vi "DQMH-GenNet Set Message Queue.vi"(8 "error in (no error)":errorcluster, 10 "Message Queue in":refnum<class "Delacor_lib_QMH_Message Queue.lvclass">, 11 "DQMH-GenNet Message Queue in":refnum<class "DQMH-GenNet Message Queue.lvclass">) -> (0 "error out":errorcluster, 3 "DQMH-GenNet Message Queue out":refnum<class "DQMH-GenNet Message Queue.lvclass">)   [LabVIEW 2014, in "hse-gennet.lvlib" / "DQMH-GenNet Message Queue.lvclass"]
doc: "Gets the message queue from the original DQMH object in <b>Message Queue in</b> and writes it to the <b>DQMH-GenNet Message Queue</b>"
uses:
  DQMH-GenNet Message Queue.lvclass
  <vilib>/Delacor/Delacor QMH/Libraries/Message Queue_class/Delacor_lib_QMH_Message Queue.lvclass
  <vilib>/Delacor/Delacor QMH/Libraries/Message Queue_class/Delacor_lib_QMH_Message Queue.lvclass/Delacor_lib_QMH_Message Queue.ctl
  <vilib>/Delacor/Delacor QMH/Libraries/Message Queue_class/Delacor_lib_QMH_Set Message Queue.vi
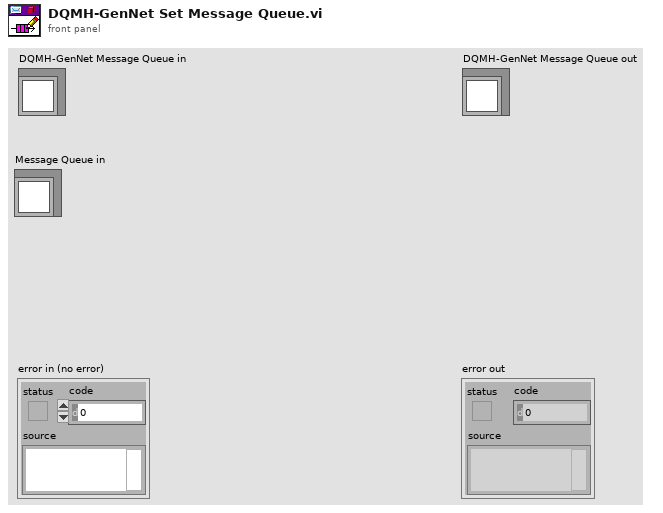
[diagram p1: front panel]
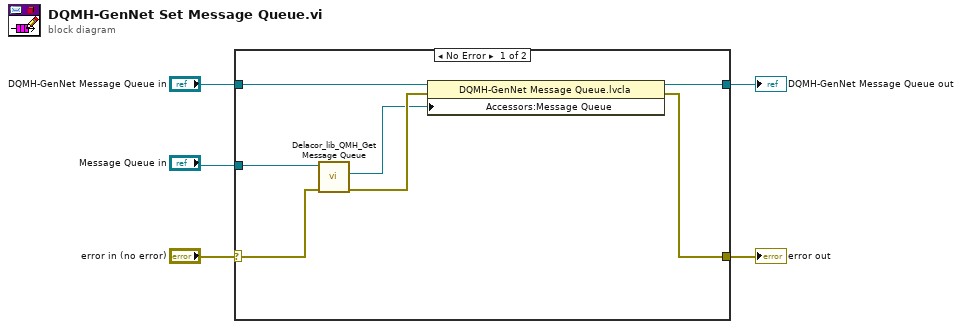
[diagram p0: block diagram]
diagram:
  n1 = case shown="No Error" "error in (no error)" {
    selector: "error in (no error)" -> [w12 w13]
    tunnel: [w7 w13] -> w4
    tunnel: [w9 w14] -> w2
    tunnel: "DQMH-GenNet Message Queue in" -> [w10 w14]
    tunnel: "Message Queue in" -> [w11 _]
    frame No Error {
      n2 = call <vilib>:"Delacor_lib_QMH_Get Message Queue.vi"("error in (no error)"=w12, "Message Queue in"=w11) -> ("error out"=w8:errorcluster, "Message Queue"=w6:refnum<queue>)  [unwired: 7 in, 1 out]
      n3 = property class="DQMH-GenNet Message Queue.lvcla"(reference=w10, error in=w8, "Accessors:Message Queue"=w6) -> (reference out=w9:refnum<class "DQMH-GenNet Message Queue.lvclass">, error out=w7:errorcluster)
    }
    frame Error {
    }
  }
  "error out" <- w4
  "DQMH-GenNet Message Queue out" <- w2
